vi "HeaderAction.vi"(0 "InstrClass":refnum<class "Calculations.lvclass"> caption="DNL_LabVIEW Object in", 11 "error in (no error)":errorcluster caption="entrée d'erreur (pas d'erreur)") -> (4 "InstrClassOut":refnum<class "Calculations.lvclass"> caption="DNL_LabVIEW Object out", 6 "DataNames":string[](array[string]), 8 "Instr Name":string, 10 "HeaderString":string, 13 "ArrDisplayNames":string[](array[string]), 14 "DisplayNames":string[](array[string]), 15 "error out":errorcluster caption="sortie d'erreur")   [LabVIEW 2019, in "Calculations.lvclass"]
uses:
  Calculations.lvclass
  C:/Programmes Labview/LabscanV1A/DevicesClass/BaseDevice/BaseDevice.lvclass
  Calculations.lvclass/Calculations.ctl
  DevicesClass/BaseDevice/BaseDevice.lvclass
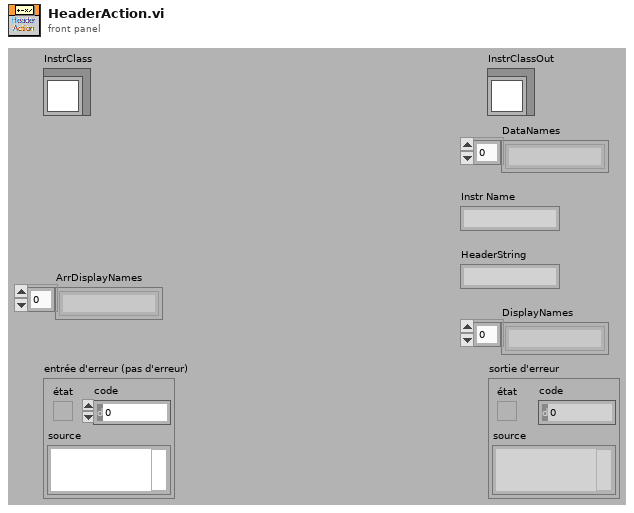
[diagram p1: front panel]
types:
  T1 = typedef "Calculations.lvclass/DefaultDev_Func.ctl" = enum16{"Multi Scan Average", "Running Average", "Summ"}
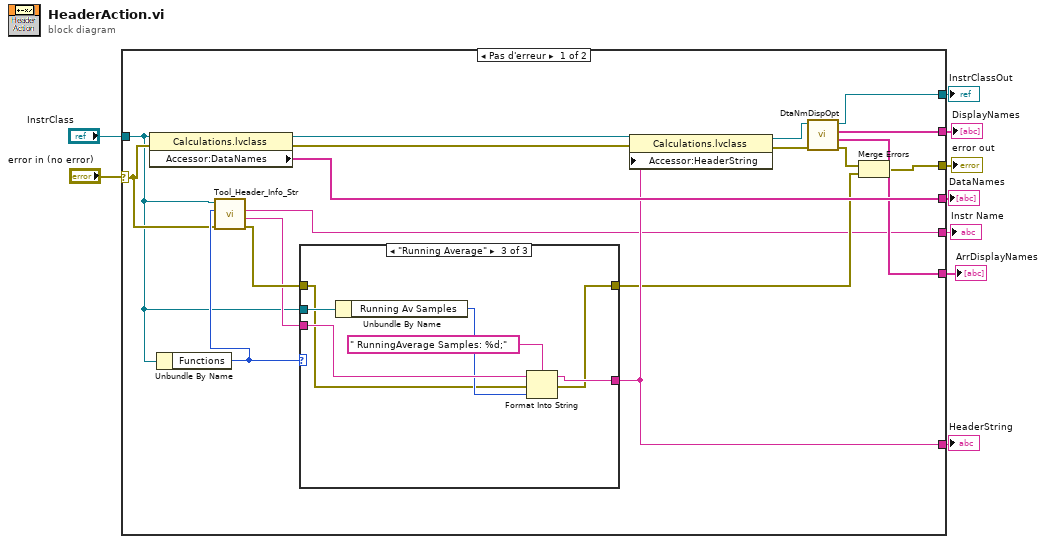
[diagram p0: block diagram]
diagram:
  n1 = case shown="Pas d'erreur" "error in (no error)" {
    selector: "error in (no error)" -> [w16 w39]
    tunnel: [w24 _] -> w8
    tunnel: [w27 _] -> w7
    tunnel: "InstrClass" -> [w10 w40]
    tunnel: [w14 w39] -> w5
    tunnel: [w21 w40] -> w3
    tunnel: [w11 _] -> w4
    tunnel: [w19 _] -> w2
    tunnel: [w18 _] -> w1
    frame No Error {
      n2 = property class="Calculations.lvclass"(reference=w10, error in=w16) -> (reference out=w26:refnum<class "Calculations.lvclass">, error out=w25:errorcluster, "Accessor:DataNames"=w27:string[])
      n3 = Unbundle By Name(w10) -> ("Functions"=w17:T1)
      n4 = call-dynamic "Tool_Header_Info_Str.vi"("error in (no error)"=w16, "Functions"=w17, "DefaultDev in"=w10) -> ("error out"=w15:errorcluster, "HdrInfoStr"=w12:string, "InstrumentName"=w11:string)  [unwired: 5 in, 1 out]
      n5 = case shown="\"Running Average\"" w17 {
        tunnel: [w28 w31 w34] -> w24
        tunnel: w15 -> [w29 w30 w33]
        tunnel: [w29 w30 w32] -> w13
        tunnel: w12 -> [w28 w31 w37]
        tunnel: w10 -> [_ _ w38]
        frame Default {
        }
        frame "Multi Scan Average" {
        }
        frame "Running Average" {
          n6 = Unbundle By Name(w38) -> ("Running Av Samples"=w36:i32)
          n7 = Format Into String(format string=" RunningAverage Samples: %d;" ("chaîne de format"), initial string=w37, error in=w33, w36) -> (resulting string=w34:string, error out=w32:errorcluster)
        }
      }
      n8 = property class="Calculations.lvclass"(reference=w26, error in=w25, "Accessor:HeaderString"=w24) -> (reference out=w20:refnum<class "Calculations.lvclass">, error out=w23:errorcluster)
      n9 = call "DtaNmDispOpt.vi"("error in (no error)"=w23, "BaseDevice en entrée"=w20) -> ("error out"=w22:errorcluster, "ArrDisplayNames"=w18:string[], "DisplayNames"=w19:string[], "BaseDevice en sortie"=w21:refnum<class "Calculations.lvclass">)  [unwired: 6 in]
      n10 = Merge Errors(w22, w13) -> (w14:errorcluster)
    }
    frame Error {
    }
  }
  "error out" <- w5
  "InstrClassOut" <- w3
  "DataNames" <- w7
  "HeaderString" <- w8
  "Instr Name" <- w4
  "DisplayNames" <- w2
  "ArrDisplayNames" <- w1
